vi "CleanHandler.ProcCases.vi"(0 "i ref in":refnum<vi>, 1 "selector":string, 2 "Data":T1, 3 "call cluster":T2={"Object"="", "Selector"="", "CallType"=enum."synchronous", "Async Object"="", "Async Selector"="", "Data Descriptor"="", "Data"=[], "Error #"=0, "Expire"=0}, 5 "error in (no error)":errorcluster) -> (14 "i ref out":refnum<vi>, 17 "answer cluster":T2={"Object"="", "Selector"="", "CallType"=enum."synchronous", "Async Object"="", "Async Selector"="", "Data Descriptor"="", "Data"=[], "Error #"=0, "Expire"=0}, 19 "error out":errorcluster)   [LabVIEW 2014, in "CleanHandler.lvlib"]
doc: "This method is called by a process from within the default case in the event loop. The methods of a class that are linked to events will be called from THIS method. Add your code here."
uses:
  CleanHandler.lvlib
  CS_Core/CSSystem/CoreDefs/CoreDefs.call_type.ctl
  CS_Core/BaseProcess/BaseProcess.descriptor string definition.ctl
  CS_Core/CSSystem/CoreDefs/CoreDefs.rawDataType.ctl
  CS_Core/CSSystem/CoreLib/CoreLib.string 2 byte array.vi
  CS_Core/CSSystem/CoreLib/CoreLib.byte array 2 double.vi
  CS_Core/CSSystem/CoreLib/CoreLib.byte array 2 int.vi
  CS_Core/BaseProcess/BaseProcess.lvlib
  CS_Core/CSSystem/CoreLib/CoreLib.lvlib
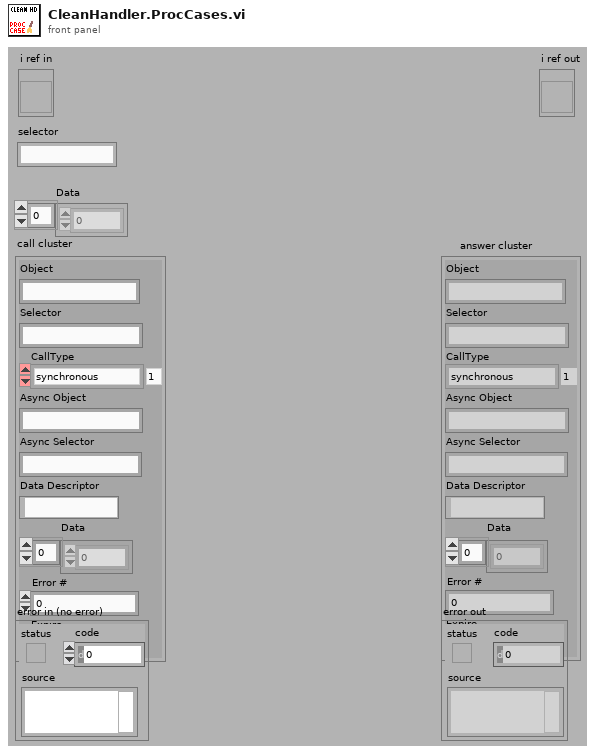
[diagram p1: front panel]
types:
  T1 = typedef "CoreDefs.rawDataType.ctl" = i8[]
  T2 = typedef "CoreDefs.call_type.ctl" = cluster{"Object":string, "Selector":string, "CallType":enum16{"simple", "synchronous", "asynchronous"}, "Async Object":string, "Async Selector":string, "Data Descriptor":T3, "Data":T1, "Error #":i32, "Expire":u32}
  T3 = typedef "BaseProcess.lvlib/BaseProcess.descriptor string definition.ctl" = string
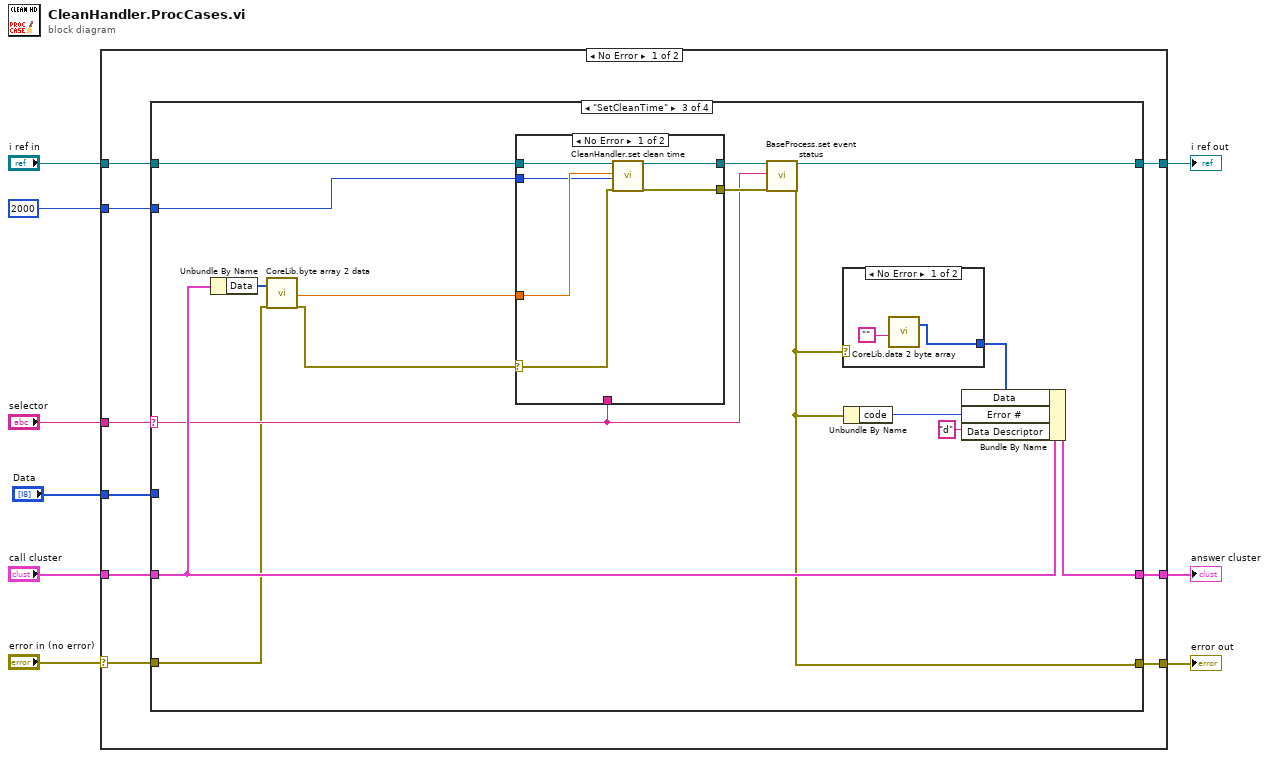
[diagram p0: block diagram]
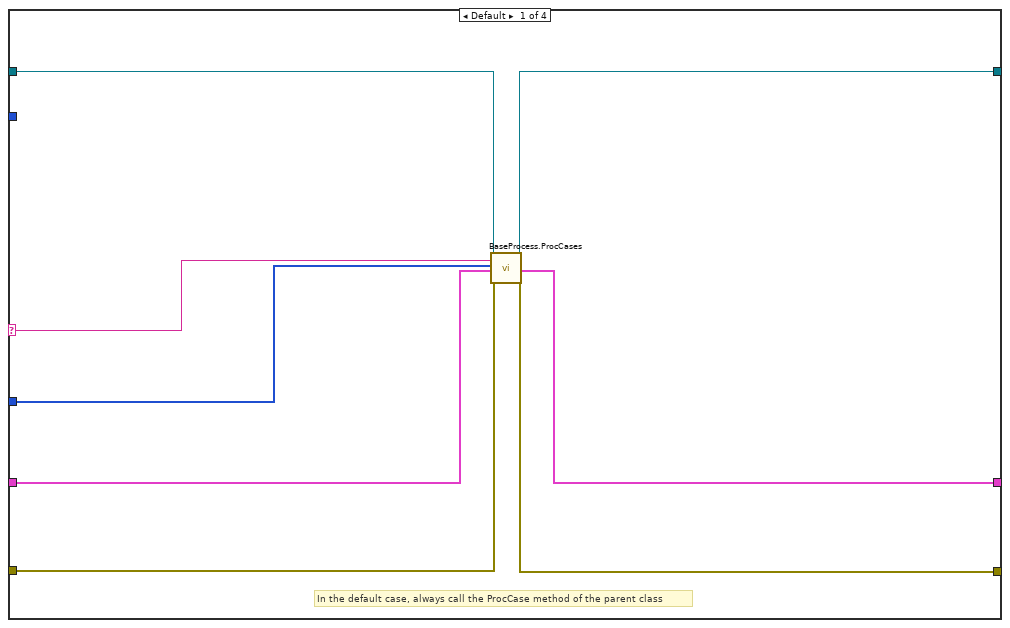
[diagram p2: hidden frame]
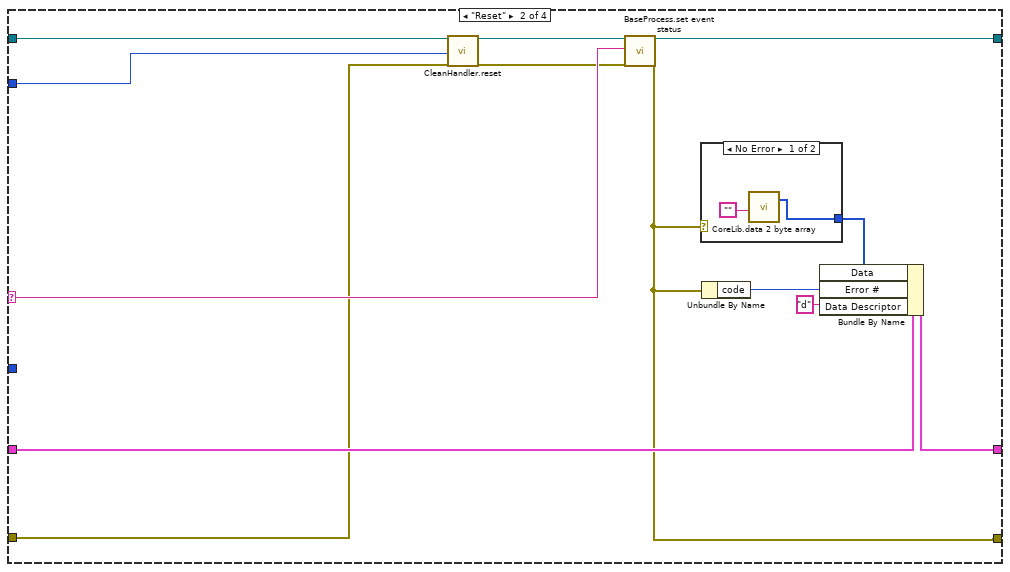
[diagram p3: hidden frame]
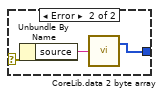
[diagram p4: hidden frame]
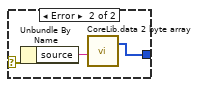
[diagram p5: hidden frame]
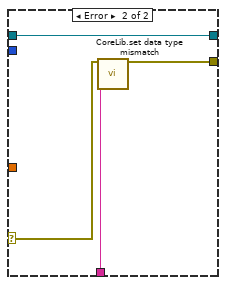
[diagram p6: hidden frame]
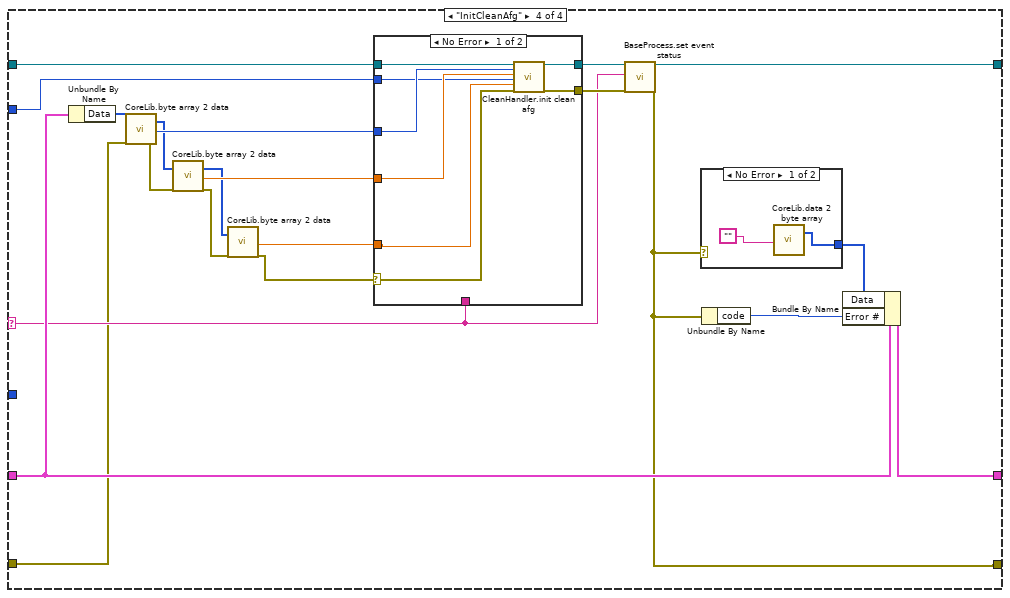
[diagram p7: hidden frame]
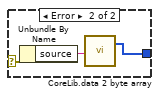
[diagram p8: hidden frame]
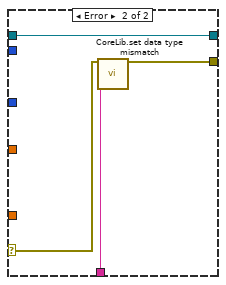
[diagram p9: hidden frame]
diagram:
  n1 = case shown="No Error" "error in (no error)" {
    selector: "error in (no error)" -> [w10 w116]
    tunnel: "selector" -> [w18 _]
    tunnel: [w17 w115] -> w8
    tunnel: "Data" -> [w16 _]
    tunnel: "call cluster" -> [w15 w115]
    tunnel: "i ref in" -> [w14 w114]
    tunnel: [w13 w114] -> w5
    tunnel: [w12 w116] -> w4
    tunnel: 2000 ("ms timeout (100)") -> [w11 _]
    frame No Error {
      n2 = case shown="\"SetCleanTime\"" w18 {
        selector: w18 -> [w20 w35 w53 w88]
        tunnel: w16 -> [w21 _ _ _]
        tunnel: w14 -> [w19 w32 w60 w96]
        tunnel: [w26 w34 w52 w87] -> w13
        tunnel: w15 -> [w22 w38 w58 w94]
        tunnel: [w23 w37 w57 w93] -> w17
        tunnel: w10 -> [w25 w30 w47 w76]
        tunnel: [w24 w36 w54 w89] -> w12
        tunnel: w11 -> [_ w28 w50 w86]
        frame Default {
          # "In the default case, always call the ProcCase method of the parent class"
          n3 = call "BaseProcess.ProcCases.vi"("i ref in"=w19, "selector"=w20, "Data"=w21, "call cluster"=w22, "error in (no error)"=w25) -> ("i ref out"=w26:refnum<vi>, "answer cluster"=w23:T2, "error out"=w24:errorcluster)  [unwired: 12 in]
        }
        frame "Reset" {
          n4 = call "CleanHandler.reset.vi"("i ref in"=w32, "ms timeout (100)"=w28, "error in (no error)"=w30) -> ("i ref out"=w31:refnum<vi>, "error out"=w29:errorcluster)  [unwired: 14 in, 1 out]
          n5 = call "BaseProcess.set event status.vi"("i ref in"=w31, "EventStatus"=w35, "error in (no error)"=w29) -> ("i ref out"=w34:refnum<vi>, "error out"=w36:errorcluster)  [unwired: 14 in, 1 out]
          n6 = case shown="No Error" w36 {
            selector: w36 -> [_ w44]
            tunnel: [w40 w42] -> w27
            frame No Error {
              n7 = call-poly "CoreLib.data 2 byte array.vi"("string"="") -> ("byteArray out"=w40:T1)  [unwired: 18 in]
            }
            frame Error {
              n8 = Unbundle By Name(w44) -> ("source"=w43:string)
              n9 = call-poly "CoreLib.data 2 byte array.vi"("string"=w43) -> ("byteArray out"=w42:T1)  [unwired: 18 in]
            }
          }
          n10 = Unbundle By Name(w36) -> ("code"=w39:i32)
          n11 = Bundle By Name(cluster=w38, "Data"=w27, "Error #"=w39, "Data Descriptor"="d") -> (w37:T2)
        }
        frame "SetCleanTime" {
          n12 = Unbundle By Name(w58) -> ("Data"=w49:T1)
          n13 = call-poly "CoreLib.byte array 2 data.vi"("byteArray"=w49, "error in (no error)"=w47) -> ("d64"=w48:dbl, "error out"=w46:errorcluster)  [unwired: 15 in, 1 out]
          n14 = case shown="No Error" w46 {
            selector: w46 -> [w66 w72]
            tunnel: [w70 w75] -> w56
            tunnel: w60 -> [w71 w75]
            tunnel: [w69 w74] -> w55
            tunnel: w53 -> [_ w73]
            tunnel: w48 -> [w68 _]
            tunnel: w50 -> [w67 _]
            frame No Error {
              n15 = call "CleanHandler.set clean time.vi"("i ref in"=w71, "clean time [s]"=w68, "ms timeout (100)"=w67, "error in (no error)"=w66) -> ("i ref out"=w70:refnum<vi>, "error out"=w69:errorcluster)  [unwired: 13 in, 1 out]
            }
            frame Error {
              n16 = call "CoreLib.set data type mismatch.vi"("error in (no error)"=w72, "error source"=w73) -> ("error out"=w74:errorcluster)  [unwired: 17 in]
            }
          }
          n17 = call "BaseProcess.set event status.vi"("i ref in"=w56, "EventStatus"=w53, "error in (no error)"=w55) -> ("i ref out"=w52:refnum<vi>, "error out"=w54:errorcluster)  [unwired: 14 in, 1 out]
          n18 = case shown="No Error" w54 {
            selector: w54 -> [_ w65]
            tunnel: [w61 w63] -> w45
            frame No Error {
              n19 = call-poly "CoreLib.data 2 byte array.vi"("string"="") -> ("byteArray out"=w61:T1)  [unwired: 18 in]
            }
            frame Error {
              n20 = Unbundle By Name(w65) -> ("source"=w64:string)
              n21 = call-poly "CoreLib.data 2 byte array.vi"("string"=w64) -> ("byteArray out"=w63:T1)  [unwired: 18 in]
            }
          }
          n22 = Unbundle By Name(w54) -> ("code"=w59:i32)
          n23 = Bundle By Name(cluster=w58, "Data"=w45, "Error #"=w59, "Data Descriptor"="d") -> (w57:T2)
        }
        frame "InitCleanAfg" {
          n24 = Unbundle By Name(w94) -> ("Data"=w85:T1)
          n25 = call-poly "CoreLib.byte array 2 data.vi"("byteArray"=w85, "error in (no error)"=w76) -> ("byteArray out"=w78:T1, "i32"=w81:i32, "error out"=w84:errorcluster)  [unwired: 15 in]
          n26 = call-poly "CoreLib.byte array 2 data.vi"("byteArray"=w78, "error in (no error)"=w84) -> ("byteArray out"=w77:T1, "d64"=w80:dbl, "error out"=w83:errorcluster)  [unwired: 15 in]
          n27 = call-poly "CoreLib.byte array 2 data.vi"("byteArray"=w77, "error in (no error)"=w83) -> ("d64"=w79:dbl, "error out"=w82:errorcluster)  [unwired: 15 in, 1 out]
          n28 = case shown="No Error" w82 {
            selector: w82 -> [w102 w110]
            tunnel: [w108 w113] -> w91
            tunnel: w96 -> [w109 w113]
            tunnel: [w107 w112] -> w90
            tunnel: w80 -> [w105 _]
            tunnel: w88 -> [_ w111]
            tunnel: w81 -> [w106 _]
            tunnel: w79 -> [w104 _]
            tunnel: w86 -> [w103 _]
            frame No Error {
              n29 = call "CleanHandler.init clean afg.vi"("i ref in"=w109, "CleanAfg"=w106, "amplitude [V]"=w105, "ms timeout (100)"=w103, "frequency [Hz]"=w104, "error in (no error)"=w102) -> ("i ref out"=w108:refnum<vi>, "error out"=w107:errorcluster)  [unwired: 11 in, 1 out]
            }
            frame Error {
              n30 = call "CoreLib.set data type mismatch.vi"("error in (no error)"=w110, "error source"=w111) -> ("error out"=w112:errorcluster)  [unwired: 17 in]
            }
          }
          n31 = call "BaseProcess.set event status.vi"("i ref in"=w91, "EventStatus"=w88, "error in (no error)"=w90) -> ("i ref out"=w87:refnum<vi>, "error out"=w89:errorcluster)  [unwired: 14 in, 1 out]
          n32 = case shown="No Error" w89 {
            selector: w89 -> [_ w101]
            tunnel: [w97 w99] -> w92
            frame No Error {
              n33 = call-poly "CoreLib.data 2 byte array.vi"("string"="") -> ("byteArray out"=w97:T1)  [unwired: 18 in]
            }
            frame Error {
              n34 = Unbundle By Name(w101) -> ("source"=w100:string)
              n35 = call-poly "CoreLib.data 2 byte array.vi"("string"=w100) -> ("byteArray out"=w99:T1)  [unwired: 18 in]
            }
          }
          n36 = Unbundle By Name(w89) -> ("code"=w95:i32)
          n37 = Bundle By Name(cluster=w94, "Data"=w92, "Error #"=w95) -> (w93:T2)
        }
      }
    }
    frame Error {
    }
  }
  "answer cluster" <- w8
  "i ref out" <- w5
  "error out" <- w4
